vi "10-Tap 8-Bit Camera with DRAM (Host).vi"() -> ()   [LabVIEW 2013]
doc: "This is the host VI for the 10-Tap 8-Bit Camera with DRAM example. This example demonstrates how to acquire images from a 10-tap, 8-bit, extended configuration, Camera Link camera and display the images on the host. This example supports area scan and line scan cameras for both continuous and finite acquisitions.\n\nThis example also demonstrates the use of DRAM as a frame buffer for very high speed acquisitions. Data packing and flow-control are also employed to maximize use of the available DRAM and FIFOs in terms of both memory space and performance.\n\nAdditionally, the example demonstrates the serial server, which allows third-party camera configuration utilities to communicate with the camera using the Camera Link serial interface while this VI is running."
uses:
  <vilib>/rvi/interface/nirviOpenFPGA/nirviOpenFPGA.xnode
  <vilib>/rvi/interface/nirviMethod/nirviMethod.xnode
  <vilib>/rvi/interface/nirviCloseFPGA/nirviCloseFPGA.xnode
  <vilib>/rvi/interface/nirviReadWriteControl/nirviReadWriteControl.xnode
  <vilib>/rvi/interface/Simulation/niFpgaSimulationCallBeginRW.vi
  <vilib>/rvi/errors/niLvFpgaAdjustHostInterfaceError.vi
  <vilib>/rvi/errors/niLvFpgaMergeErrorWithErrorCode.vi
  <vilib>/FPGAPlugInAG/Dynamic/niLvFpga_Reset_Dynamic.vi
  <vilib>/FPGAPlugInAG/Dynamic/niLvFpga_Run_Dynamic.vi
  FPGA Bitfiles/10-Tap8-BitCamer_PXIe-7965R_10-Tap8-BitCamer_5A7595F4.lvbitx
  Program Files (x86)/National Instruments/LabVIEW 2013/examples/FlexRIO/IO Modules/NI 1483/10-Tap 8-bit Camera with DRAM/10-Tap 8-Bit Camera with DRAM (FPGA).vi
  <vilib>/FPGAPlugInAG/Dynamic/niLvFpga_StartFifo_Dynamic.vi
  <vilib>/FPGAPlugInAG/Dynamic/niLvFpga_Close_Dynamic.vi
  <vilib>/FPGAPlugInAG/Dynamic/niLvFpga_ConfigureFifo_Dynamic.vi
  <vilib>/FPGAPlugInAG/Dynamic/niLvFpga_ReadFifo_Dynamic.vi
  <vilib>/userdefined/High Color/nirio_resource_hc.ctl
panel:
  in  "DMA Buffer Size\n(In Images)":u32=64 caption="DMA Buffer Size"
  in  "Signal Mapping":T1(ring)=enum."Basler 10-tap"
  out "Acq In Progress":bool
  in  "Line Scan":bool
  in  "Frames To Acquire":u32=1 caption="Frames To Acquire\n(0 = infinite)"
  in  "Cancel":bool
  out "Acq'd Frame Width":u32
  in  "Stopped":bool
  in  "RIO Device":T2="RIO0"
  out "DMA Write Timeout":bool
  out "Module Enabled":bool
  in  "Start Serial Server":bool=TRUE
  out "Frames Acq'd":u32
  out "Acq'd Frame Height":u32
  out "Image":T3(plugin-control)
  in  "Acquire":bool
  in  "Stop":bool
  in  "Image Height":u32=1024 max=65535
  in  "Image Width":u32=1280 max=65535 step=40
  out "Initialized":bool
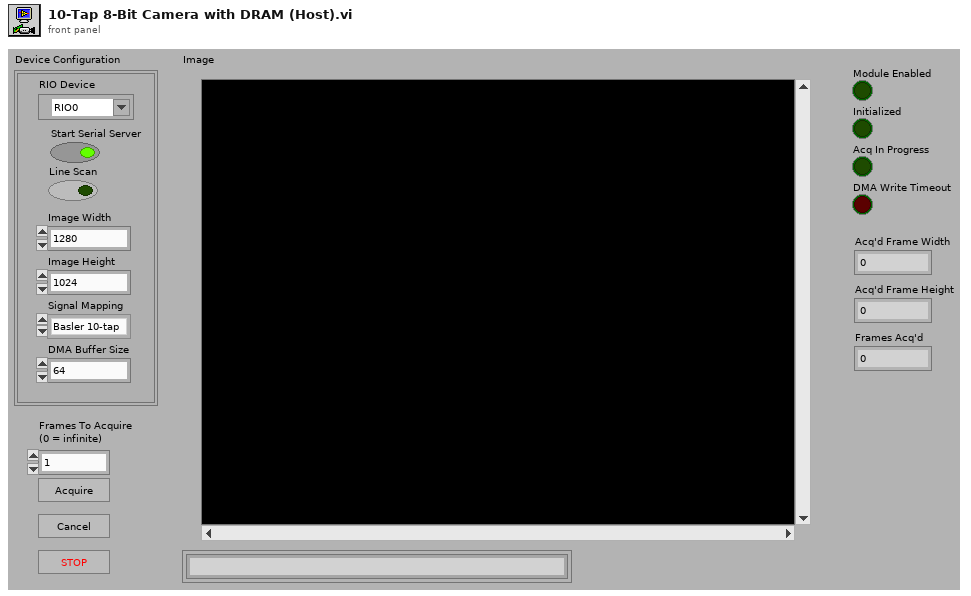
[diagram p1: front panel]
types:
  T1 = enum8{"Standard", "Basler 10-tap", "Vosskühler 10-tap"}
  T2 = typedef "nirio_resource_hc.ctl" = tag
  T3 = typedef "IMAQ Image.ctl" = refnum<image>
  T4 = typedef "Image Type" = u32
  T5 = enum16{"big-endian, network order", "native, host order", "little-endian"}
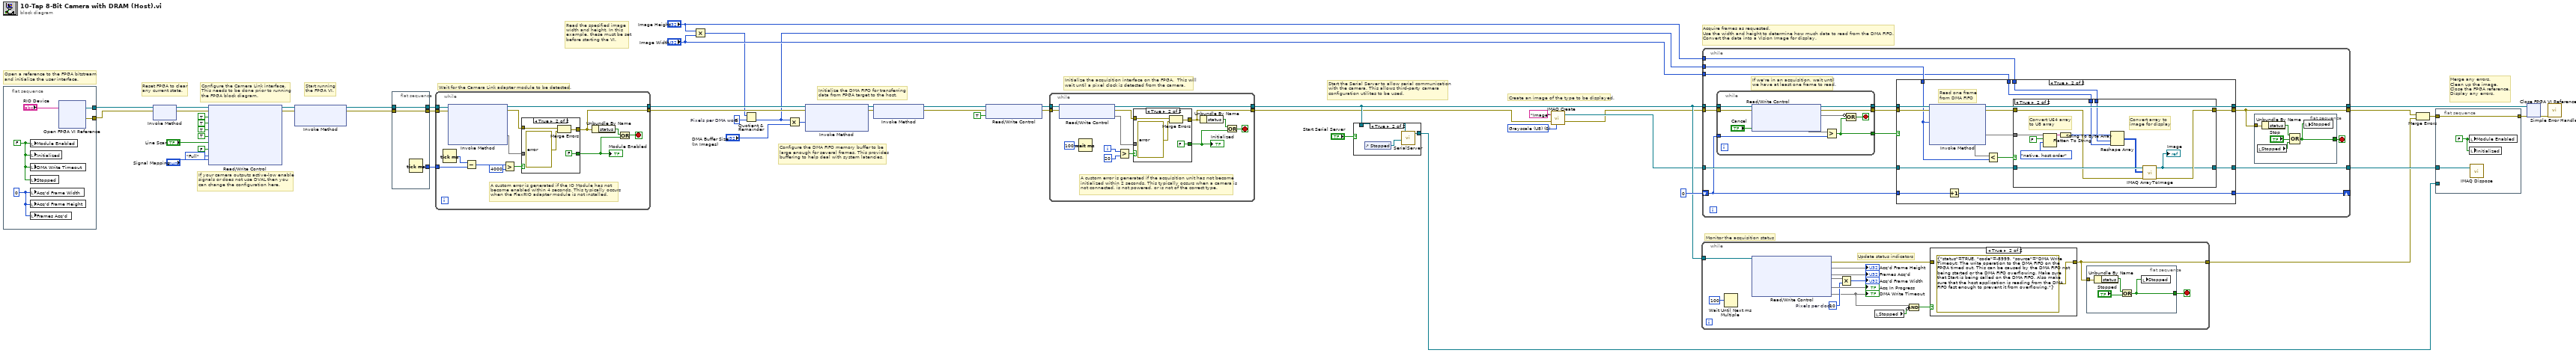
[diagram p0: block diagram]
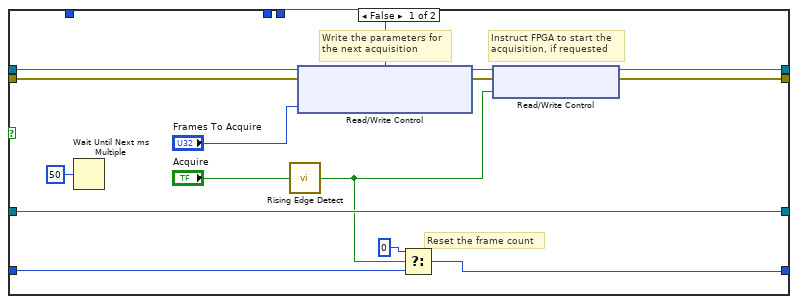
[diagram p4: hidden frame]
diagram:
  w3 = u32 8  # Pixels per DMA word
  w47 = T4 0 items=["Grayscale (U8)", "Grayscale (I16)", "Grayscale (SGL)", "Complex (CSG)", "RGB (U32)", "HSL (U32)", "RGB (U64)", "Grayscale (U16)"] ("Image Type")
  # "If your camera outputs active-low enable\nsignals or does not use DVAL then you \ncan change the configuration here."
  # "Configure the DMA FIFO memory buffer to be\nlarge enough for several frames. This provides\nbuffering to help deal with system latencies."
  # "Start running\nthe FPGA VI."
  # "Reset FPGA to clear\nany current state."
  # "Read the specified image\nwidth and height. In this\nexample, these must be set\nbefore starting the VI."
  # "Merge any errors.\nClean up the image.\nClose the FPGA reference.\nDisplay any errors."
  # "Acquire frames as requested.\nUse the width and height to determine how much data to read from the DMA FIFO.\nConvert the data into a Vision Image for display."
  # "Monitor the acquisition status"
  # "Start the Serial Server to allow serial communication\nwith the camera. This allows third-party camera\nconfiguration utilites to be used."
  # "Create an image of the type to be displayed."
  # "Initialize the acquisition interface on the FPGA.  This will\nwait until a pixel clock is detected from the camera."
  # "Wait for the Camera Link adapter module to be detected."
  # "Initialize the DMA FIFO for transferring\ndata from FPGA target to the host."
  # "Configure the Camera Link interface.\nThis needs to be done prior to running\nthe FPGA block diagram."
  # "Open a reference to the FPGA bitstream\nand initialize the user interface."
  n1 = flat-sequence {
    tunnel: [w53] -> w38
    tunnel: [w52] -> w51
    frame #0 {
      w56 = u32 0 ("Num Lines Acq'd")
      w55 = FALSE ("stop")
      n2 = local write "Module Enabled"(w55) -> ()
      n3 = local write "Initialized"(w55) -> ()
      n4 = local write "DMA Write Timeout"(w55) -> ()
      n5 = local write "Stopped"(w55) -> ()
      n6 = local write "Acq'd Frame Width"(w56) -> ()
      n7 = local write "Acq'd Frame Height"(w56) -> ()
      n8 = local write "Frames Acq'd"(w56) -> ()
      n9 = xnode "Open FPGA VI Reference"("resource name"="RIO Device") -> ("FPGA VI Reference Out"=w53:refnum<k20>, "error out"=w52:errorcluster)  [unwired: 1 in]
    }
  }
  n10 = xnode "Invoke Method"("FPGA VI Reference In"=w38, "error in"=w51) -> ("FPGA VI Reference Out"=w25:refnum<k20>, "error out"=w28:errorcluster)
  n11 = xnode "Read/Write Control"("FPGA VI Reference In"=w25, "error in"=w28, "CL Config.FVAL Active High"=TRUE ("IO Module Config.CL FVAL Active High"), "CL Config.LVAL Active High"=TRUE ("IO Module Config.CL LVAL Active High"), "CL Config.DVAL Active High"=TRUE ("IO Module Config.CL DVAL Active High"), "CL Config.Spare Active High"=TRUE ("IO Module Config.CL Spare Active High"), "CL Config.Line Scan"="Line Scan", "Acq Control.Ignore DVAL"=FALSE ("CL Config.Line Scan"), "CL Config.Configuration"=enum8{"Base", "Medium", "Full"}."Full", "CL Config.Signal Mapping"="Signal Mapping") -> ("FPGA VI Reference Out"=w29:refnum<k20>, "error out"=w27:errorcluster)
  n12 = xnode "Invoke Method"("FPGA VI Reference In"=w29, "error in"=w27) -> ("FPGA VI Reference Out"=w10:refnum<k20>, "error out"=w15:errorcluster)  [unwired: 1 in]
  n13 = flat-sequence {
    tunnel: [w59] -> w18
    tunnel: w10 -> [w58]
    tunnel: [w58] -> w17
    tunnel: [w57] -> w16
    tunnel: w15 -> [w57]
    frame #0 {
      n14 = Tick Count (ms)() -> (millisecond timer value=w59:u32)
    }
  }
  n15 = while {
    tunnel: w17 -> [w73]
    tunnel: [w72] -> w37
    tunnel: w16 -> [w71]
    tunnel: [w65] -> w36
    tunnel: w18 -> [w60]
    stop <- w69 stop-if-true
    # "A custom error is generated if the IO Module has not\nbecome enabled within 4 seconds. This typically occurs\nwhen the FlexRIO adapter module is not installed."
    n16 = Tick Count (ms)() -> (millisecond timer value=w63:u32)
    n17 = xnode "Invoke Method"("FPGA VI Reference In"=w73, "error in"=w71) -> ("FPGA VI Reference Out"=w72:refnum<k20>, "error out"=w67:errorcluster, "I/O Enabled?"=w64)  [unwired: 3 out]
    n18 = Subtract(x=w63, y=w60) -> (x-y=w62:u32)
    n19 = Greater?(x=w62, y=u32 4000) -> (0:w68:bool)
    n20 = case shown="True" w68 {
      tunnel: [w75 FALSE] -> w66
      tunnel: w64 -> [w75 _]
      tunnel: w67 -> [w74 w77]
      tunnel: [w74 w79] -> w65
      frame False {
      }
      frame True {
        n21 = Merge Errors(w77, errorcluster {"status"=TRUE, "code"=-8999, "source"="IO Module Status: The IO Module did not initialize before the specified timeout. This typically occurs when the FlexRIO adapter module is not properly connected to the FlexRIO FPGA module."} ("error in")) -> (w79:errorcluster)
      }
    }
    "Module Enabled" <- w66
    n22 = Unbundle By Name(w65) -> ("status"=w70:bool)
    n23 = Or(x=w70, y=w66) -> (x .or. y?=w69:bool)
  }
  n24 = Multiply(x="Image Height", y="Image Width") -> (x*y=w2:u32)
  n25 = Quotient & Remainder(x=w2, y=w3) -> (floor(x/y)=w1:u32)  [unwired: 1 out]
  n26 = Multiply(x=w1, y="DMA Buffer Size\n(In Images)") -> (x*y=w19:u32)
  n27 = xnode "Invoke Method"("FPGA VI Reference In"=w37, "error in"=w36, "Requested Depth"=w19) -> ("FPGA VI Reference Out"=w35:refnum<k20>, "error out"=w34:errorcluster)  [unwired: 1 out]
  n28 = xnode "Invoke Method"("FPGA VI Reference In"=w35, "error in"=w34) -> ("FPGA VI Reference Out"=w20:refnum<k20>, "error out"=w33:errorcluster)
  n29 = xnode "Read/Write Control"("FPGA VI Reference In"=w20, "error in"=w33, "Acq Control.Initialize"=TRUE ("Arm Acquisition")) -> ("FPGA VI Reference Out"=w50:refnum<k20>, "error out"=w49:errorcluster)
  n30 = while {
    tunnel: w50 -> [w87]
    tunnel: w49 -> [w86]
    tunnel: [w85] -> w12
    tunnel: [w89] -> w11
    i -> [w81]
    stop <- w92 stop-if-true
    # "A custom error is generated if the acquisition unit has not become\ninitialized within 2 seconds. This typically occurs when a camera is\nnot connected, is not powered, or is not of the correct type."
    n31 = xnode "Read/Write Control"("FPGA VI Reference In"=w87, "error in"=w86) -> ("FPGA VI Reference Out"=w85:refnum<k20>, "error out"=w84:errorcluster, "Acq Status.Initialized"=w83)
    n32 = Wait (ms)(milliseconds to wait=u32 100) -> ()  [unwired: 1 out]
    n33 = Greater?(x=w81, y=20) -> (0:w82:bool)
    n34 = case shown="True" w82 {
      tunnel: [w94 FALSE] -> w88
      tunnel: w83 -> [w94 _]
      tunnel: w84 -> [w93 w96]
      tunnel: [w93 w98] -> w89
      frame False {
      }
      frame True {
        n35 = Merge Errors(w96, errorcluster {"status"=TRUE, "code"=-8999, "source"="Acquisition Initialization: This error typically occurs when a camera is not properly connected, is not powered, or is not of the correct type."} ("error in")) -> (w98:errorcluster)
      }
    }
    "Initialized" <- w88
    n36 = Unbundle By Name(w89) -> ("status"=w91:bool)
    n37 = Or(x=w91, y=w88) -> (x .or. y?=w92:bool)
  }
  n38 = case shown="True" "Start Serial Server" {
    tunnel: [_ w99] -> w39
    tunnel: w12 -> [_ w100]
    frame False {
    }
    frame True {
      n39 = control-ref of="Stopped"() -> (w101:refnum<vi>)
      n40 = call "SerialServer.vi"("Stop Refnum"=w101, "FPGA VI Reference In"=w100) -> ("FPGA VI Reference Out"=w99:refnum<k20>)  [unwired: 5 in]
    }
  }
  n41 = call "IMAQ Create"("Image Name"="Image", "Image Type"=w47, "error in (no error)"=w11) -> ("New Image"=w7:T3, "error out"=w6:errorcluster)  [unwired: 2 in]
  n42 = while {
    tunnel: w12 -> [w112]
    tunnel: [w115] -> w30
    stop <- w114 stop-if-true
    w105 = u32 10  # Pixels per clock
    # "Update status indicators"
    n43 = Wait Until Next ms Multiple(millisecond multiple=u32 100) -> ()  [unwired: 1 out]
    n44 = xnode "Read/Write Control"("FPGA VI Reference In"=w112) -> ("error out"=w111:errorcluster, "Acq Status.Lines Per Frame"=→"Acq'd Frame Height", "Acq Status.Frames Acq'd"=→"Frames Acq'd", "Acq Status.Clocks Per Line"=w106, "Acq Status.Acq In Progress"=→"Acq In Progress", "Acq Status.DMA Write Timeout"=w103)  [unwired: 1 in, 1 out]
    "DMA Write Timeout" <- w103
    n45 = Multiply(x=w106, y=w105) -> (x*y=→"Acq'd Frame Width":u32)
    n46 = local read "Stopped"() -> (w102:bool)
    n47 = Compound Arithmetic op=AND(w103, invert w102) -> (w104:bool)
    n48 = case shown="True" w104 {
      tunnel: w111 -> [w120 _]
      tunnel: [w120 errorcluster {"status"=TRUE, "code"=-8999, "source"="DMA Write Timeout: The write operation to the DMA FIFO on the FPGA timed out. This can be caused by the DMA FIFO not being started or the DMA FIFO overflowing. Make sure that Start is being called on the DMA FIFO. Also make sure that the host application is reading from the DMA FIFO fast enough to prevent it from overflowing."} ("error out")] -> w115
      frame False {
      }
      frame True {
      }
    }
    n49 = flat-sequence {
      tunnel: w115 -> [w119]
      tunnel: [w117] -> w114
      frame #0 {
        n50 = Unbundle By Name(w119) -> ("status"=w118:bool)
        n51 = Or(x=w118, y="Stopped") -> (x .or. y?=w117:bool)
        n52 = local write "Stopped"(w117) -> ()
      }
    }
  }
  n53 = while {
    tunnel: w12 -> [w128]
    tunnel: w6 -> [w127]
    tunnel: w1 -> [w136]
    tunnel: "Image Height" -> [w135]
    tunnel: "Image Width" -> [w134]
    tunnel: w7 -> [w133]
    tunnel: [w131] -> w31
    tunnel: [w132] -> w46
    tunnel: [w129] -> w41
    shift-right: [w123] -> _
    shift-left: u32 0 -> [w122]
    stop <- w130 stop-if-true
    # "If we're in an acquisition, wait until\nwe have at least one frame to read."
    n54 = while {
      tunnel: w128 -> [w143]
      tunnel: w127 -> [w142]
      tunnel: [w140] -> w126
      tunnel: [w141] -> w125
      tunnel: w122 -> [w146]
      tunnel: [w144] -> w124
      stop <- w145 stop-if-true
      n55 = xnode "Read/Write Control"("FPGA VI Reference In"=w143, "error in"=w142, "Acq Control.Cancel Acq"="Cancel") -> ("FPGA VI Reference Out"=w141:refnum<k20>, "error out"=w140:errorcluster, "Acq Status.Acq In Progress"=w139, "Acq Status.Frames Acq'd"=w138)
      n56 = Greater?(x=w138, y=w146) -> (0:w144:bool)
      n57 = Compound Arithmetic op=OR(invert w139, w144) -> (w145:bool)
    }
    n58 = case shown="True" w124 {
      tunnel: w125 -> [w162 w174]
      tunnel: w126 -> [w161 w173]
      tunnel: w136 -> [_ w167]
      tunnel: w135 -> [w155 w181]
      tunnel: w134 -> [_ w180]
      tunnel: w133 -> [w166 w179]
      tunnel: [w157 w177] -> w131
      tunnel: [w160 w176] -> w132
      tunnel: [w166 w175] -> w129
      tunnel: w122 -> [w163 w172]
      tunnel: [w165 w171] -> w123
      frame False {
        # "Reset the frame count"
        # "Instruct FPGA to start the\nacquisition, if requested"
        # "Write the parameters for\nthe next acquisition"
        n59 = Wait Until Next ms Multiple(millisecond multiple=u32 50) -> ()  [unwired: 1 out]
        n60 = call "Rising Edge Detect.vi"("Input"="Acquire") -> ("Pulse"=w152:bool)  [unwired: 4 in]
        n61 = xnode "Read/Write Control"("FPGA VI Reference In"=w162, "error in"=w161, "Acq Control.Line Scan Height"=w155, "Acq Control.Frames To Acq"="Frames To Acquire") -> ("FPGA VI Reference Out"=w159:refnum<k20>, "error out"=w158:errorcluster)
        n62 = Select(t=u32 0, s=w152, f=w163) -> (s? t:f=w165:u32)
        n63 = xnode "Read/Write Control"("FPGA VI Reference In"=w159, "error in"=w158, "Acq Control.Acquire"=w152) -> ("FPGA VI Reference Out"=w160:refnum<k20>, "error out"=w157:errorcluster)
      }
      frame True {
        # "Read one frame\nfrom DMA FIFO"
        n64 = xnode "Invoke Method"("FPGA VI Reference In"=w174, "error in"=w173, "Number of Elements"=w167) -> ("FPGA VI Reference Out"=w176:refnum<k20>, "error out"=w178:errorcluster, "Data"=w170:void[], "Elements Remaining"=w168)  [unwired: 1 in]
        n65 = Increment(x=w172) -> (x+1=w171:u32)
        n66 = Less?(x=w168, y=w167) -> (x < y?=w169:bool)
        n67 = case shown="True" w169 {
          tunnel: w181 -> [_ w195]
          tunnel: w180 -> [_ w194]
          tunnel: w179 -> [w183 w193]
          tunnel: w178 -> [w182 w192]
          tunnel: [w182 w191] -> w177
          tunnel: [w183 w190] -> w175
          tunnel: w170 -> [_ w187]
          frame False {
            # "Do not display the image if we're falling behind in the acquisition."
          }
          frame True {
            # "Convert U64 array\nto U8 array"
            # "Convert array to\nimage for display"
            n68 = Flatten To String(anything=w187, prepend array or string size? (T)=FALSE, byte order (0:big-endian, network order)=T5."native, host order") -> (data string=w185:string)  [unwired: 1 in, 2 out]
            n69 = String To Byte Array(string=w185) -> (unsigned byte array=w184:u8[])
            n70 = Reshape Array(w184, w195, w194) -> (w189:u8[][])
            n71 = call "IMAQ ArrayToImage"("error in (no error)"=w192, "Image Pixels (U8)"=w189, "Image"=w193) -> ("error out"=w191:errorcluster, "Image Out"=w190:T3)  [unwired: 7 in]
            "Image" <- w190
          }
        }
      }
    }
    n72 = flat-sequence {
      tunnel: w131 -> [w149]
      tunnel: [w148] -> w130
      frame #0 {
        n73 = local read "Stopped"() -> (w147:bool)
        n74 = Unbundle By Name(w149) -> ("status"=w150:bool)
        n75 = Compound Arithmetic op=OR(w150, "Stop", w147) -> (w148:bool)
        n76 = local write "Stopped"(w148) -> ()
      }
    }
  }
  n77 = Merge Errors(w31, w30) -> (w32:errorcluster)
  n78 = flat-sequence {
    tunnel: w32 -> [w197]
    tunnel: [w197] -> w43
    tunnel: w41 -> [w198]
    tunnel: w39 -> [_]
    frame #0 {
      w196 = FALSE ("Module Enabled")
      n79 = local write "Module Enabled"(w196) -> ()
      n80 = local write "Initialized"(w196) -> ()
      n81 = call "IMAQ Dispose"("Image"=w198) -> ()  [unwired: 5 in, 1 out]
    }
  }
  n82 = xnode "Close FPGA VI Reference"("FPGA VI Reference In"=w46, "error in"=w43) -> ("error out"=w40:errorcluster)
  n83 = call <vilib>:"Simple Error Handler.vi"("error in (no error)"=w40) -> ()  [unwired: 4 in, 5 out]
